vi "Get Train Rate.vi"(10 "going up?":bool=TRUE, 11 "Power Supply in":refnum<class "Power Supply.lvclass">) -> (2 "Rate Out":dbl[unit]=0.11666666666666667, 3 "Power Supply Out":refnum<class "Power Supply.lvclass">)   [LabVIEW 2015, in "Power Supply.lvclass"]
uses:
  Power Supply.lvclass
  Power Supply.lvclass/Power Supply.ctl
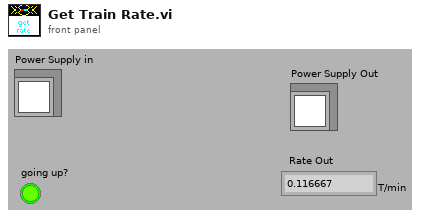
[diagram p1: front panel]
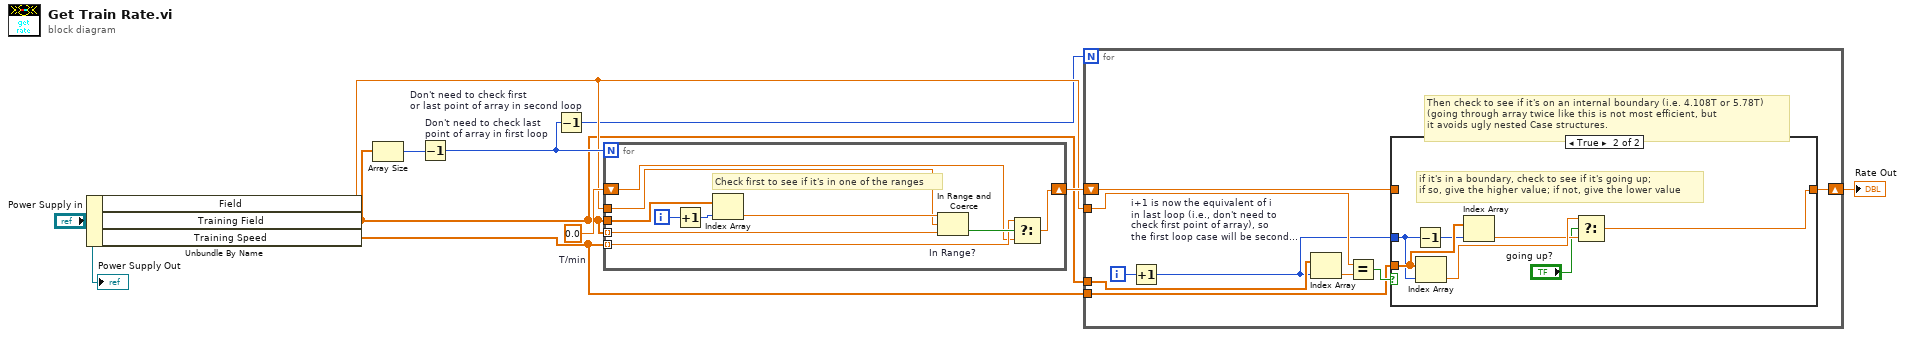
[diagram p0: block diagram]
diagram:
  w8 = dbl[unit] 0.0  # T/min
  n1 = Unbundle By Name("Power Supply in") -> ("Field"=w4:dbl[unit], "Training Field"=w3:dbl[unit][], "Training Speed"=w2:dbl[unit][])
  n2 = Array Size(array=w3) -> (size(s)=w9:i32)
  n3 = Decrement "Don't need to check last \npoint of array in first loop"(x=w9) -> (x-1=w5:i32)
  n4 = Decrement "Don't need to check first\nor last point of array in second loop"(x=w5) -> (x-1=w1:i32)
  n5 = for {
    N: w5 -> [_]
    tunnel: w4 -> [w17]
    tunnel: w3 -> [w16]
    tunnel: w3 -> [w15] mode=indexing
    tunnel: w2 -> [w13] mode=indexing
    shift-right: [w12] -> w7
    shift-left: w8 -> [w11]
    i -> [w18]
    # "Check first to see if it's in one of the ranges"
    n6 = Increment(x=w18) -> (x+1=w19:i32)
    n7 = Index Array(array=w16, index=w19) -> (element=w20:dbl[unit])
    n8 = In Range and Coerce "In Range?"(upper limit=w20, x=w17, lower limit=w15) -> (In Range?=w14:bool)  [unwired: 1 out]
    n9 = Select(t=w13, s=w14, f=w11) -> (s? t:f=w12:dbl[unit])
  }
  n10 = for {
    N: w1 -> [_]
    tunnel: w4 -> [w26]
    tunnel: w3 -> [w24]
    tunnel: w2 -> [w22]
    shift-right: [w28] -> w6
    shift-left: w7 -> [w27]
    i -> [w29]
    # "Then check to see if it's on an internal boundary (i.e. 4.108T or 5.78T)\n(going through array twice like this is not most efficient, but\nit avoids ugly nested Case structures."
    n11 = Increment "i+1 is now the equivalent of i\nin last loop (i.e., don't need to \ncheck first point of array), so \nthe first loop case will be second\npoint"(x=w29) -> (x+1=w21:i32)
    n12 = Index Array(array=w24, index=w21) -> (element=w23:dbl[unit])
    n13 = Equal?(x=w26, y=w23) -> (x = y?=w25:bool)
    n14 = case shown="True" w25 {
      tunnel: [w30 w37] -> w28
      tunnel: w27 -> [w30 _]
      tunnel: w22 -> [_ w36]
      tunnel: w21 -> [_ w34]
      frame False {
        # "if not at a boundary, just use the value determined \nfrom the range business of the last loop"
      }
      frame True {
        # "if it's in a boundary, check to see if it's going up; \nif so, give the higher value; if not, give the lower value"
        n15 = Decrement(x=w34) -> (x-1=w35:i32)
        n16 = Index Array(array=w36, index=w34) -> (element=w33:dbl[unit])
        n17 = Index Array(array=w36, index=w35) -> (element=w32:dbl[unit])
        n18 = Select(t=w33, s="going up?", f=w32) -> (s? t:f=w37:dbl[unit])
      }
    }
  }
  "Rate Out" <- w6
  "Power Supply Out" <- "Power Supply in"
